vi "FRCts20_EspEngine_FormatArrayOfKeysInts.vi"(8 "error IO":errorcluster, 9 "Values":i32[](array[numeric]), 10 "KeyBaseName":string, 11 "httpRequestID":u32) -> (0 "error IO":errorcluster, 3 "httpRequestID out":u32)   [LabVIEW 2013, in "FRCts20_EspEngine.lvlib"]
uses:
  FRCts20_EspEngine.lvlib
  <vilib>/wsapi/subVIs/Set Integer ESP Variable.vi
  <vilib>/wsapi/NI_WebServices.lvlib
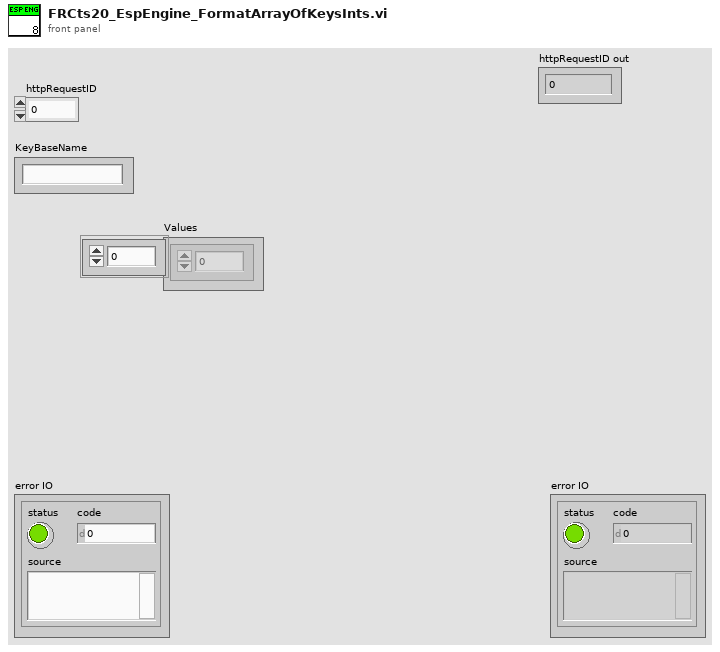
[diagram p1: front panel]
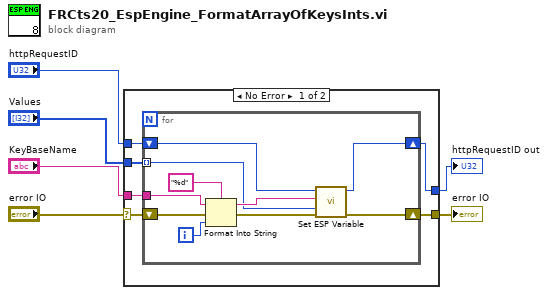
[diagram p0: block diagram]
diagram:
  n1 = case shown="No Error" "error IO" {
    selector: "error IO" -> [w12 w23]
    tunnel: [w8 w23] -> w6
    tunnel: "Values" -> [w11 _]
    tunnel: "httpRequestID" -> [w10 _]
    tunnel: [w9 _] -> w2
    tunnel: "KeyBaseName" -> [w7 _]
    frame No Error {
      n2 = for {
        tunnel: w11 -> [w14] mode=indexing
        tunnel: w7 -> [w22]
        shift-right: [w16] -> w9
        shift-left: w10 -> [w17]
        shift-right: [w15] -> w8
        shift-left: w12 -> [w19]
        i -> [w21]
        n3 = Format Into String(format string="%d", initial string=w22, error in=w19, w21) -> (resulting string=w18:string, error out=w13:errorcluster)
        n4 = call-poly <vilib>:"Set ESP Variable.vi"("error in (no error)"=w13, "value"=w14, "key"=w18, "httpRequestID"=w17) -> ("error out"=w15:errorcluster, "httpRequestID out"=w16:u32)  [unwired: 6 in]
      }
    }
    frame Error {
    }
  }
  "error IO" <- w6
  "httpRequestID out" <- w2
